vi "CAN Frame to Data.vi"(8 "Fehler (Eingang)":errorcluster, 9 "Messdaten in":dbl[](array[numeric]), 10 "selected SAE J-1939 Signals":refnum<k21>[](array[refnum]), 11 "CAN Daten aktuell":T1[](array[typedef]) {"payload" format="%x"; "timestamp" format="%<%.7X\n%x>T"; "type" items=["CAN Data"=0, "CAN Remote"=1, "CAN Bus Error"=2, "CAN 2.0 Data"=8, "CAN FD Data"=16, "CAN FD+BRS Data"=24, "J1939 Data"=192, "Delay"=224, "Log Trigger"=225, "Start Trigger"=226]; "identifier" format="%x"}) -> (0 "Fehler (Ausgang)":errorcluster, 1 "Messdaten out":dbl[](array[numeric]), 2 "FrameNames":string[](array[string]), 4 "SignalNames":string[](array[string]))   [LabVIEW 2020]
uses:
  <resource>/objmgr/xnet.rc
  CAN Konfig.lvlib
  <vilib>/xnet/xnet.llb/XNET Create Session (Conversion).vi
  <vilib>/xnet/xnet.llb/XNET Convert (Frame CAN to Signal).vi
  <vilib>/xnet/xnet.llb/XNET Frame Type CAN.ctl
  <vilib>/xnet/xnet.llb/XNET Frame CAN.ctl
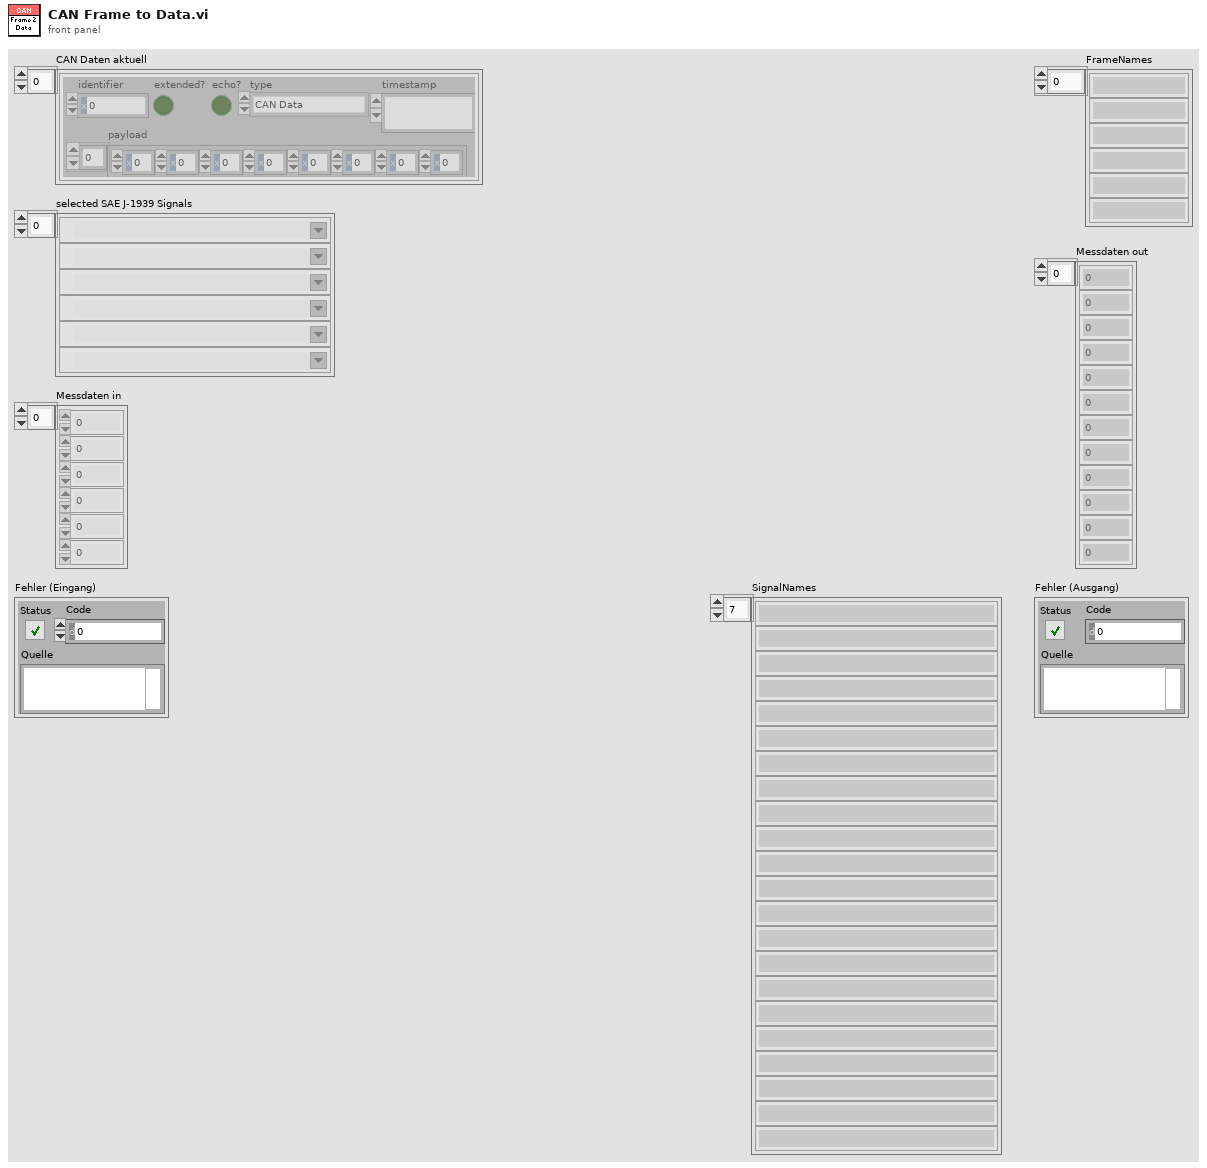
[diagram p1: front panel]
types:
  T1 = typedef "XNET Frame CAN.ctl" = cluster{"timestamp":timestamp, "payload":u8[], "identifier":u32, "type":T2, "extended?":bool, "echo?":bool}
  T2 = typedef "XNET Frame Type CAN.ctl" = u8
  T3 = enum16{"lesen", "schreiben", "laden", "speichern"}
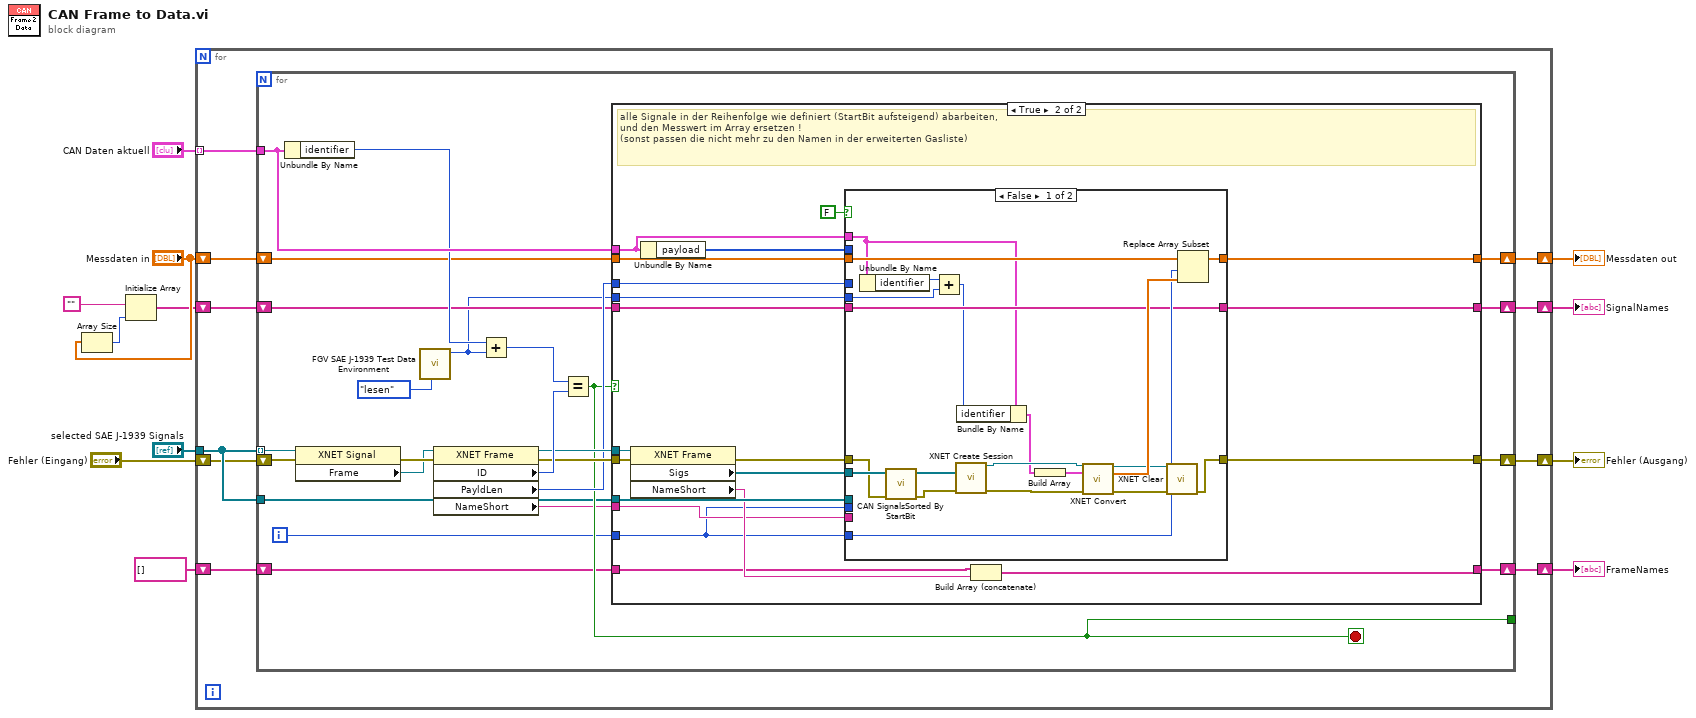
[diagram p0: block diagram]
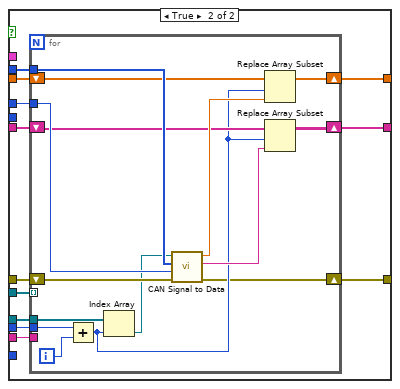
[diagram p3: hidden frame]
diagram:
  n1 = Array Size(array="Messdaten in") -> (size(s)=w6:i32)
  n2 = Initialize Array("", w6) -> (w4:string[])
  n3 = for {
    tunnel: "selected SAE J-1939 Signals" -> [w20]
    tunnel: "CAN Daten aktuell" -> [w22] mode=indexing
    shift-right: [w19] -> w10
    shift-left: string[] [] ("NameShort") -> [w17]
    shift-right: [w18] -> w9
    shift-left: "Messdaten in" -> [w21]
    shift-right: [w15] -> w3
    shift-left: w4 -> [w16]
    shift-right: [w14] -> w2
    shift-left: "Fehler (Eingang)" -> [w13]
    n4 = for {
      tunnel: w20 -> [w46] mode=indexing
      tunnel: w22 -> [w40]
      shift-right: [w35] -> w18
      shift-left: w21 -> [w34]
      tunnel: [w33] -> _
      tunnel: w20 -> [w32]
      shift-right: [w29] -> w19
      shift-left: w17 -> [w30]
      shift-right: [w27] -> w15
      shift-left: w16 -> [w28]
      shift-right: [w25] -> w14
      shift-left: w13 -> [w24]
      i -> [w31]
      stop <- w33 stop-if-true
      n5 = Unbundle By Name(w40) -> ("identifier"=w38:u32)
      n6 = property class="XNET Signal"(reference=w46, error in=w24) -> (error out=w45:errorcluster, "Frame"=w44:refnum<k21>)  [unwired: 1 out]
      n7 = call "FGV SAE J-1939 Test Data Environment.vi"("Aktion"=T3."lesen") -> ("Offset Frame ID"=w23:i32)  [unwired: 7 in, 3 out]
      n8 = property class="XNET Frame"(reference=w44, error in=w45) -> (reference out=w42:refnum<k21>, error out=w41:errorcluster, "ID"=w43:u32, "PayldLen"=w36:u32, "NameShort"=w26:string)
      n9 = Add(x=w38, y=w23) -> (x+y=w37:u32)
      n10 = Equal?(x=w37, y=w43) -> (x = y?=w33:bool)
      n11 = case shown="True" w33 {
        tunnel: w42 -> [_ w70]
        tunnel: w41 -> [w47 w69]
        tunnel: w40 -> [_ w53]
        tunnel: w36 -> [_ w68]
        tunnel: [w50 w56] -> w35
        tunnel: w34 -> [w50 w65]
        tunnel: w31 -> [_ w55]
        tunnel: w32 -> [_ w67]
        tunnel: [w49 w62] -> w29
        tunnel: w30 -> [w49 w63]
        tunnel: w28 -> [w48 w61]
        tunnel: [w48 w60] -> w27
        tunnel: w26 -> [_ w57]
        tunnel: [w47 w59] -> w25
        tunnel: w23 -> [_ w51]
        frame False {
          # "immer gleiche Anzahl an Messwerten wie selektierte Signale\n(ausgewählte SAE J-1938 Kanäle)"
        }
        frame True {
          # "alle Signale in der Reihenfolge wie definiert (StartBit aufsteigend) abarbeiten,\nund den Messwert im Array ersetzen !\n(sonst passen die nicht mehr zu den Namen in der erweiterten Gasliste)"
          n12 = property class="XNET Frame"(reference=w70, error in=w69) -> (error out=w58:errorcluster, "Sigs"=w54:refnum<k21>[], "NameShort"=w64:string)  [unwired: 1 out]
          n13 = Unbundle By Name(w53) -> ("payload"=w66:u8[])
          n14 = case shown="False" FALSE {
            tunnel: w68 -> [_ w102]
            tunnel: w67 -> [_ w101]
            tunnel: w66 -> [_ w100]
            tunnel: w65 -> [w79 w99]
            tunnel: w61 -> [w80 w98]
            tunnel: [w80 w97] -> w60
            tunnel: [w71 w96] -> w59
            tunnel: w58 -> [w81 w95]
            tunnel: w57 -> [_ w94]
            tunnel: w54 -> [w82 w93]
            tunnel: [w83 w92] -> w56
            tunnel: w55 -> [_ w91]
            tunnel: w55 -> [w84 _]
            tunnel: w53 -> [w77 _]
            tunnel: w51 -> [w75 _]
            frame False {
              n15 = Unbundle By Name(w77) -> ("identifier"=w76:u32)
              n16 = call "CAN SignalsSorted By StartBit.vi"("Fehler (Eingang, kein Fehler)"=w81, "selected SAE J-1939 Signals"=w82) -> ("Fehler (Ausgang)"=w88:errorcluster, "sorted selected SAE J-1939 Signals"=w86:refnum<k21>[])  [unwired: 8 in]
              n17 = Add(x=w76, y=w75) -> (x+y=w74:u32)
              n18 = call-poly <vilib>:"XNET Create Session.vi"("signal list"=w86, "error in (no error)"=w88) -> ("session out"=w87:refnum<k21>, "error out"=w89:errorcluster)  [unwired: 12 out]
              n19 = Bundle By Name(cluster=w77, "identifier"=w74) -> (w78:T1)
              n20 = Build Array(w78) -> (w85:T1[])
              n21 = call-poly <vilib>:"XNET Convert.vi"("session in"=w87, "frame data"=w85, "error in (no error)"=w89) -> ("session out"=w73:refnum<k21>, "signal data"=w90:dbl[], "error out"=w72:errorcluster)  [unwired: 10 in]
              n22 = call <vilib>:"XNET Clear.vi"("session in"=w73, "error in (no error)"=w72) -> ("error out"=w71:errorcluster)  [unwired: 13 in]
              n23 = Replace Array Subset(array=w79, new element=w90, index=w84) -> (w83:dbl[])
            }
            frame True {
              n24 = for {
                tunnel: w93 -> [_] mode=indexing
                tunnel: w102 -> [w110]
                tunnel: w100 -> [w117]
                tunnel: w101 -> [w116]
                tunnel: w91 -> [w115]
                shift-right: [w112] -> w92
                shift-left: w99 -> [w111]
                shift-right: [w106] -> w97
                shift-left: w98 -> [w109]
                shift-right: [w105] -> w96
                shift-left: w95 -> [w104]
                tunnel: w94 -> [_]
                i -> [w114]
                n25 = Add(x=w115, y=w114) -> (x+y=w107:i32)
                n26 = Index Array(array=w116, index=w107) -> (element=w103:refnum<k21>)
                n27 = call "CAN Signal to Data.vi"("Fehler (Eingang, kein Fehler)"=w104, "PayldLen"=w110, "payload"=w117, "Referenz (Eingang)"=w103) -> ("Fehler (Ausgang)"=w105:errorcluster, "NameShort"=w108:string, "value"=w113:dbl)  [unwired: 5 in]
                n28 = Replace Array Subset(array=w111, new element=w113, index=w107) -> (w112:dbl[])
                n29 = Replace Array Subset(array=w109, new element=w108, index=w107) -> (w106:string[])
              }
            }
          }
          n30 = Build Array (concatenate)(w63, w64) -> (w62:string[])
        }
      }
    }
  }
  "Messdaten out" <- w9
  "FrameNames" <- w10
  "SignalNames" <- w3
  "Fehler (Ausgang)" <- w2
